vi "Set Initialization Data - ModuleA.vi"(8 "error in":errorcluster, 11 "MainUI in":refnum<class "MainUI.lvclass">) -> (0 "error out":errorcluster, 3 "MainUI out":refnum<class "MainUI.lvclass">)   [LabVIEW 2024, in "MainUI.lvclass"]
doc: "In this VI you can set the initialization data of a statically-linked subWorker."
uses:
  MainUI.lvclass
  ModuleA/Initialization Data.ctl
  ModuleA/Response Cases.ctl
  <vilib>/addons/_Workers/Library/Case Label.ctl
  MainUI.lvclass/MainUI.ctl
  ModuleA/ModuleA.lvclass
  C:/Program Files (x86)/National Instruments/LabVIEW 2024/vi.lib/addons/_Workers/Library/Classes/Worker/Worker.lvclass
  <vilib>/addons/_Workers/Library/Workers.lvlib
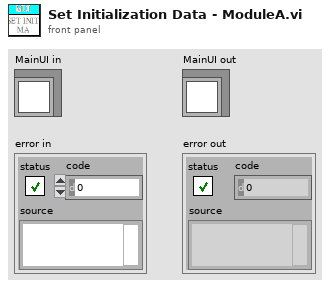
[diagram p1: front panel]
types:
  T1 = typedef "ModuleA.lvclass/Initialization Data.ctl" = cluster{"Response Cases":T2}
  T2 = typedef "ModuleA.lvclass/Response Cases.ctl" = cluster{"Placeholder - Can be deleted":string, "FeedbackMA_Data":T3}
  T3 = typedef "Workers.lvlib/Case Label.ctl" = string
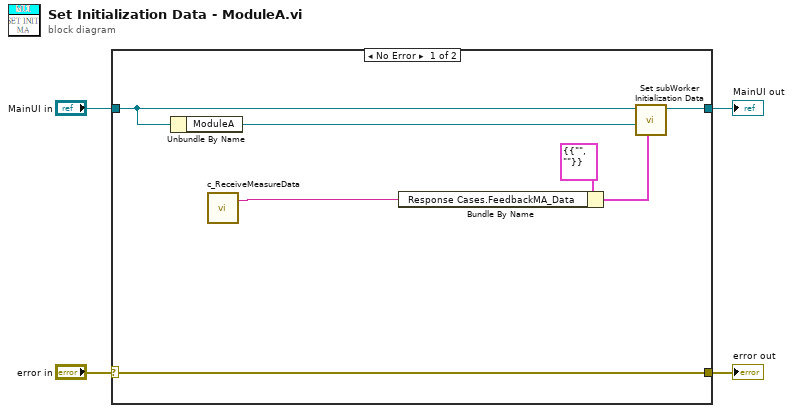
[diagram p0: block diagram]
diagram:
  n1 = case shown="No Error" "error in" {
    selector: "error in" -> [w11 w13]
    tunnel: [w11 w13] -> w3
    tunnel: [w9 w12] -> w2
    tunnel: "MainUI in" -> [w8 w12]
    frame No Error {
      n2 = Unbundle By Name(w8) -> ("ModuleA"=w10:refnum<class "ModuleA.lvclass">)
      n3 = call "c_ReceiveMeasureData.vi"() -> ("Case Label"=w5:T3)  [unwired: 1 in]
      n4 = Bundle By Name(cluster=T1 {"Response Cases"={"Placeholder - Can be deleted"="", "FeedbackMA_Data"=""}} ("Initialization Data"), "Response Cases.FeedbackMA_Data"=w5) -> (w6:T1)
      n5 = call-dynamic "Set subWorker Initialization Data.vi"("Initialization Data"=w6, "subWorker"=w10, "Worker"=w8) -> ("Worker out"=w9:refnum<class "MainUI.lvclass">)  [unwired: 8 in]
    }
    frame Error {
    }
  }
  "error out" <- w3
  "MainUI out" <- w2
